vi "Mining and Dumping_r3.vi"() -> ()   [LabVIEW 2015]
uses:
  <vilib>/myRIO/Instrument Drivers/Onboard IO/PWM/typedefs/PWM Reference.ctl
  <vilib>/myRIO/Common/Instrument Driver Framework/Utilities/typedefs/myRIO Generic Hardware Reference.ctl
  <vilib>/myRIO/Common/Instrument Driver Framework/Utilities/typedefs/Hardware Version Enum.ctl
  <vilib>/myRIO/Common/Instrument Driver Framework/Utilities/typedefs/myRIO v1.0 Reference.ctl
  <vilib>/myRIO/Common/Instrument Driver Framework/Utilities/typedefs/Generic FPGA Reference.ctl
  <vilib>/myRIO/Common/Instrument Driver Framework/myRIO v1.0/PWM/typedefs/PWM Channels Enum.ctl
  <vilib>/myRIO/Instrument Drivers/Onboard IO/PWM/typedefs/PWM Configuration.ctl
  <vilib>/userdefined/High Color/nirio_resource_hc.ctl
  <vilib>/myRIO/Instrument Drivers/Onboard IO/AI/typedefs/AI Reference.ctl
  <vilib>/myRIO/Common/Instrument Driver Framework/myRIO v1.0/AI/typedefs/AI Channels List.ctl
  <vilib>/myRIO/Common/Instrument Driver Framework/myRIO v1.0/AI/typedefs/AI Channels Enum.ctl
  <vilib>/myRIO/Common/Instrument Driver Framework/Utilities/typedefs/Analog Scaling Constants List.ctl
  <vilib>/myRIO/Common/Instrument Driver Framework/Utilities/typedefs/Analog Scaling Constants.ctl
  <vilib>/myRIO/Common/Instrument Driver Framework/Utilities/vis/Is FPGA Ref Available.vi
  <vilib>/myRIO/Common/Instrument Driver Framework/myRIO v1.0/AI/vis/myRIO v1.1 Open AI.vi
  <vilib>/myRIO/Instrument Drivers/Onboard IO/AI/vis/Read.vi
  <vilib>/myRIO/Common/Instrument Driver Framework/myRIO v1.0/PWM/vis/myRIO v1.1 Open PWM.vi
  <vilib>/myRIO/Instrument Drivers/Onboard IO/PWM/vis/Set Duty Cycle and Frequency.vi
  <vilib>/myRIO/Common/Instrument Driver Framework/Utilities/vis/Validate Channels.vi
  <vilib>/myRIO/Common/Instrument Driver Framework/myRIO v1.0/AI/vis/myRIO v1.0 Reserve AI.vi
  <vilib>/myRIO/Common/Instrument Driver Framework/myRIO v1.0/PWM/vis/myRIO v1.0 Reserve PWM.vi
  <vilib>/myRIO/Common/Instrument Driver Framework/myRIO v1.0/AI/vis/myRIO v1.0 Build MUX Configuration AI.vi
  <vilib>/myRIO/Common/Instrument Driver Framework/myRIO v1.0/Resource Manager/vis/myRIO v1.0 Reserve Channel List.vi
  <vilib>/myRIO/Common/Instrument Driver Framework/myRIO v1.0/PWM/vis/myRIO v1.0 Build MUX Configuration PWM.vi
  <vilib>/myRIO/Common/Instrument Driver Framework/myRIO v1.0/Resource Manager/vis/myRIO v1.0 Reserve Channel.vi
  <vilib>/myRIO/Common/Instrument Driver Framework/myRIO v1.0/Resource Manager/vis/myRIO v1.0 Unreserve Channel.vi
  <vilib>/myRIO/Common/Instrument Driver Framework/myRIO v1.0/Resource Manager/vis/myRIO v1.0 Create Configuration List.vi
  <vilib>/myRIO/Common/Instrument Driver Framework/myRIO v1.0/Resource Manager/vis/myRIO v1.0 Build Mutex Name.vi
  <vilib>/Utility/VariantDataType/GetNumericInfo.vi
  <vilib>/Utility/error.llb/Error Cluster From Error Code.vi
  <vilib>/myRIO/Common/Instrument Driver Framework/myRIO v1.0/myRIO v1.1 Open.vi
  <vilib>/myRIO/Common/Instrument Driver Framework/Utilities/vis/IO Manager.vi
  <vilib>/myRIO/Common/Instrument Driver Framework/Utilities/vis/Configuration Manager.vi
  <vilib>/myRIO/Common/Instrument Driver Framework/myRIO v1.0/Resource Manager/vis/myRIO v1.0 Configure IO.vi
  <vilib>/myRIO/Common/Instrument Driver Framework/myRIO v1.0/myRIO v1.0 Close.vi
  <vilib>/myRIO/Common/Instrument Driver Framework/myRIO v1.0/PWM/vis/myRIO v1.0 Write PWM.vi
  <vilib>/myRIO/Common/Instrument Driver Framework/myRIO v1.0/AI/vis/myRIO v1.0 Get Scaling Constants AI.vi
  <vilib>/myRIO/Common/Instrument Driver Framework/myRIO v1.0/AI/vis/myRIO v1.0 Read AI.vi
  <vilib>/myRIO/Express VI/Onboard IO/PWM/PWM Express VI.xnode
  <vilib>/myRIO/Instrument Drivers/Onboard IO/PWM/vis/myRIO PWM Open.xnode
  <vilib>/myRIO/Express VI/Onboard IO/AI/AI Express VI.xnode
  <vilib>/myRIO/Instrument Drivers/Onboard IO/AI/vis/myRIO AI Open.xnode
  <vilib>/myRIO/Instrument Drivers/Onboard IO/PWM/PWM.lvlib
  <vilib>/myRIO/Instrument Drivers/Onboard IO/AI/AI.lvlib
panel:
  in  "Mine or Dump":i16
  out "Stop":bool
  out "Elapsed Time (s)":dbl
  out "Elapsed Time (s) 2":dbl caption="Elapsed Time (s)"
  out "Stop Dumping":bool
  out "Servo Positioin 2":dbl
  out "Servo Position 1":dbl
  out "Servo Stop":i64
  out "Stop Mining":bool
  out "DRUM IS FULL":bool
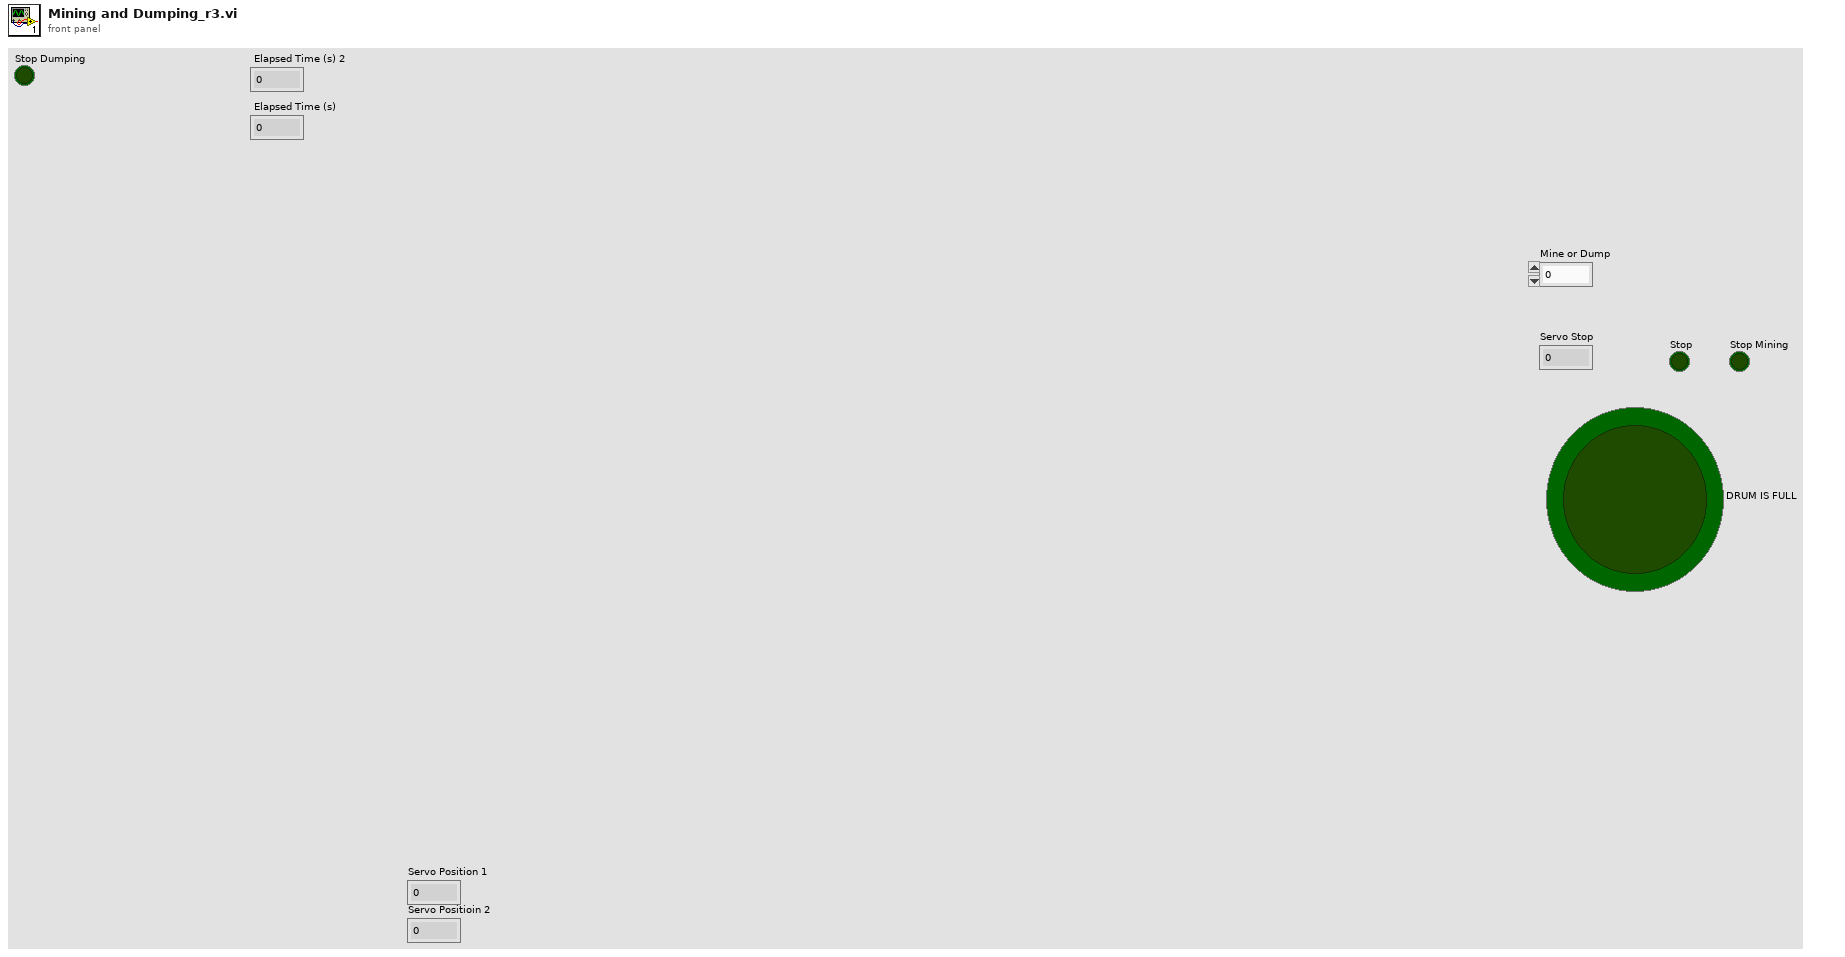
[diagram p1: front panel]
types:
  T1 = typedef "PWM.lvlib/PWM Reference.ctl" = cluster{"myRIO Reference":T2, "PWM Channels Enum":T6, "PWM Configuration":T7}
  T2 = typedef "myRIO Generic Hardware Reference.ctl" = cluster{"myRIO Model":T3, "myRIO Hardware Reference":T4}
  T3 = typedef "Hardware Version Enum.ctl" = enum16{"Unknown", "myRIO-1900", "myRIO-1950", "roboRIO"}
  T4 = typedef "myRIO v1.0 Reference.ctl" = cluster{"Generic FPGA Reference":T5, "Allow multiple opens":bool}
  T5 = typedef "Generic FPGA Reference.ctl" = refnum<k20>
  T6 = typedef "PWM Channels Enum.ctl" = enum16{"Not Connected", "C/PWM0", "C/PWM1", "A/PWM0", "A/PWM1", "A/PWM2", "B/PWM0", "B/PWM1", "B/PWM2", "PWM/PWM0", "PWM/PWM1", "PWM/PWM2", "PWM/PWM3", "PWM/PWM4", "PWM/PWM5", "PWM/PWM6", "PWM/PWM7", "PWM/PWM8", "PWM/PWM9"}
  T7 = typedef "PWM.lvlib/PWM Configuration.ctl" = cluster{"Frequency":dbl, "Duty Cycle":dbl}
  T8 = typedef "nirio_resource_hc.ctl" = tag
  T9 = typedef "AI.lvlib/AI Reference.ctl" = cluster{"myRIO Reference":T2, "AI Channels List":T10, "AI Scaling Constants List":T12}
  T10 = typedef "AI Channels List.ctl" = T11[]
  T11 = typedef "AI Channels Enum.ctl" = enum16{"Not Connected", "AudioIn/Left", "AudioIn/Right", "C/AI0", "C/AI1", "A/AI0", "A/AI1", "A/AI2", "A/AI3", "B/AI0", "B/AI1", "B/AI2", "B/AI3", "AI/AI0", "AI/AI1", "AI/AI2", "AI/AI3"}
  T12 = typedef "Analog Scaling Constants List.ctl" = T13[]
  T13 = typedef "Analog Scaling Constants.ctl" = cluster{"LSB Weight (Volts)":dbl, "Offset (Volts)":dbl, "Signed?":bool}
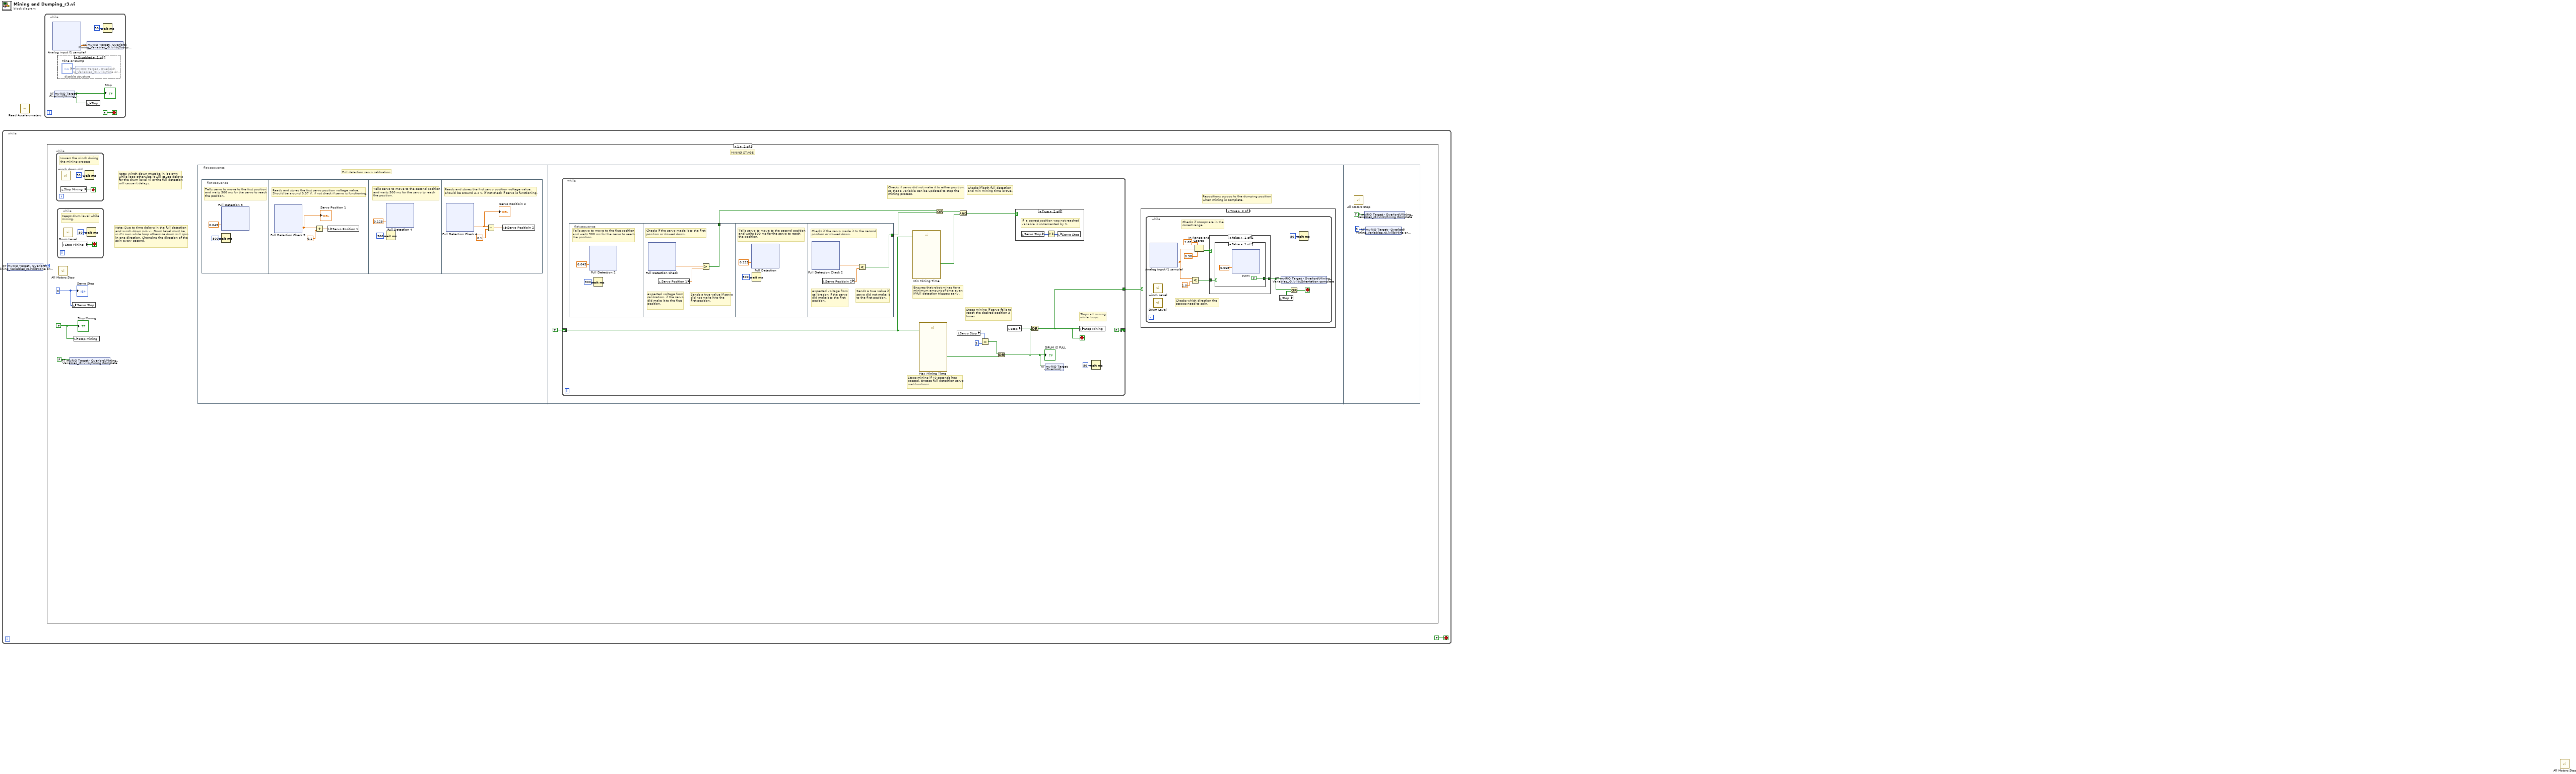
[diagram p0: block diagram]
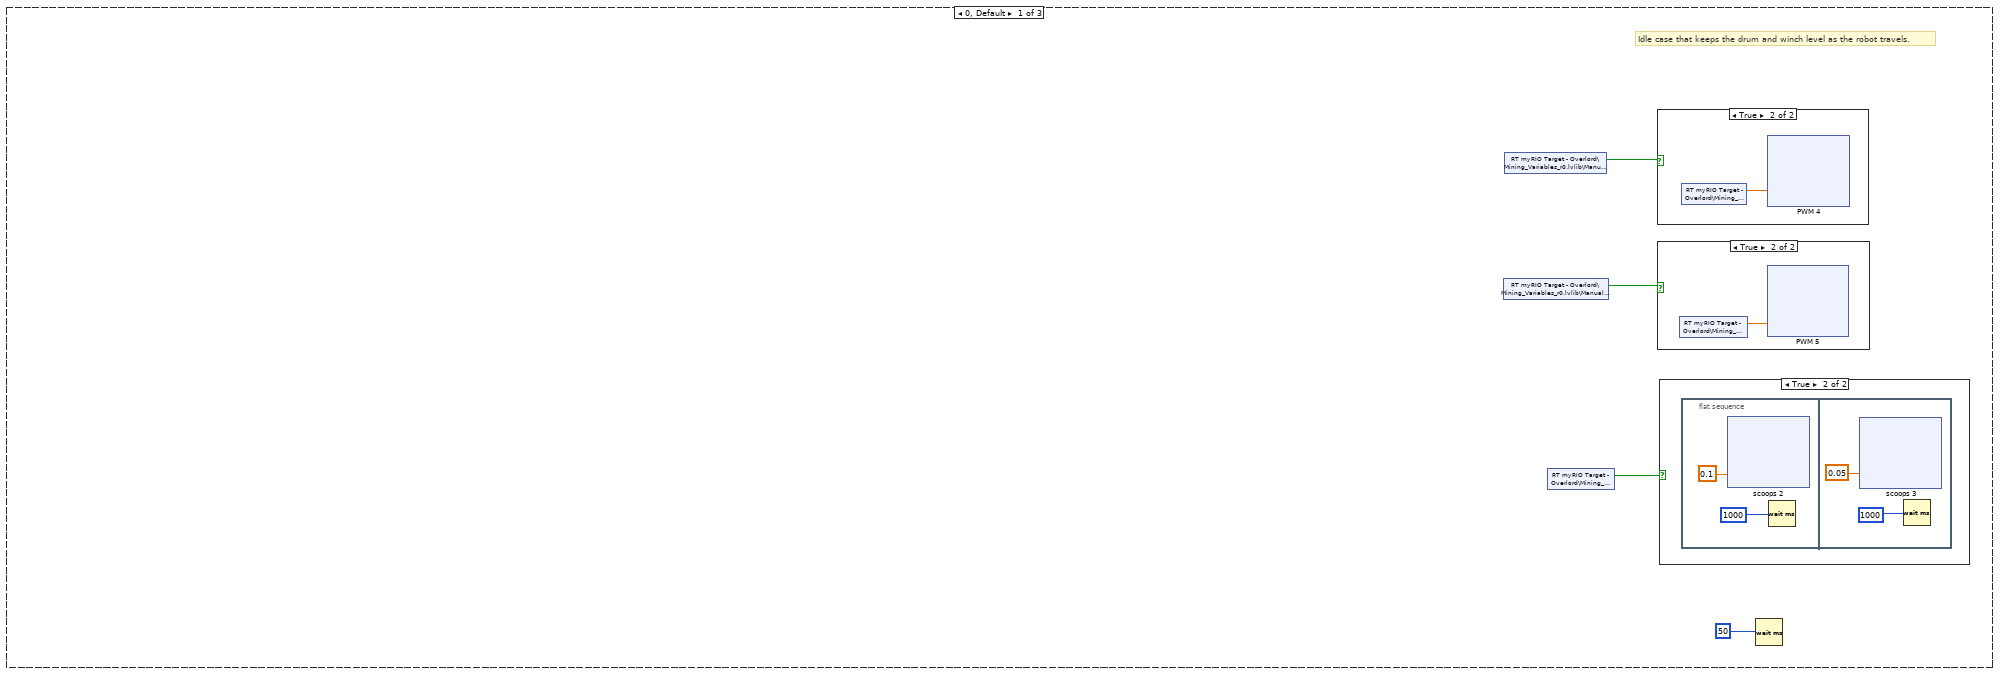
[diagram p3: hidden frame]
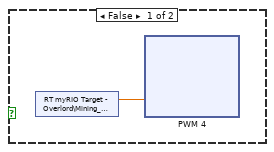
[diagram p4: hidden frame]
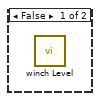
[diagram p5: hidden frame]
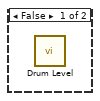
[diagram p6: hidden frame]
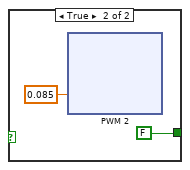
[diagram p8: hidden frame]
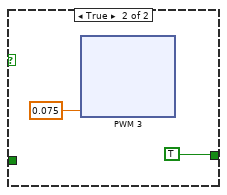
[diagram p9: hidden frame]
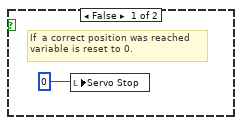
[diagram p10: hidden frame]
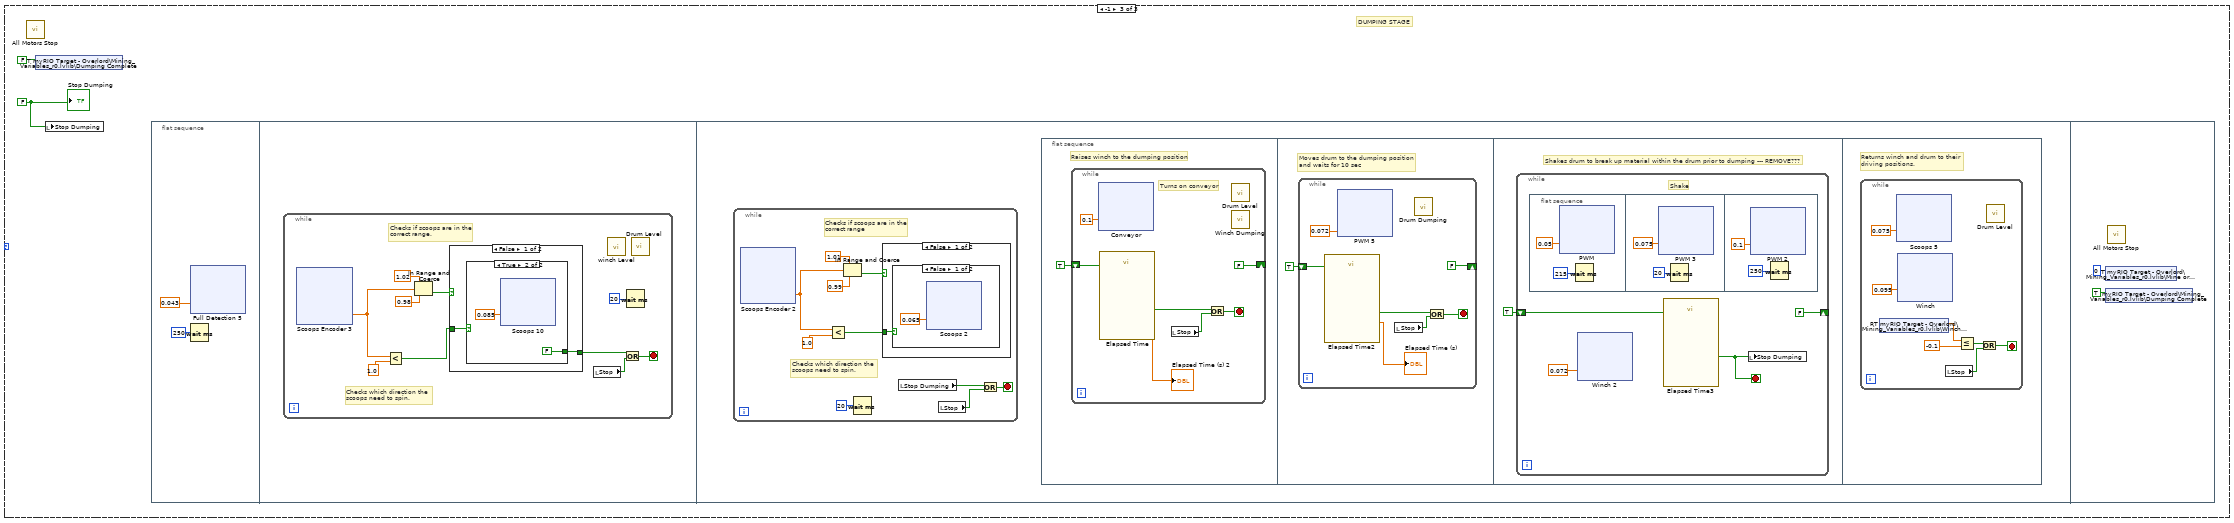
[diagram p11: hidden frame]
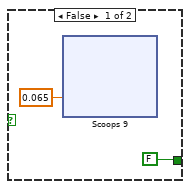
[diagram p12: hidden frame]
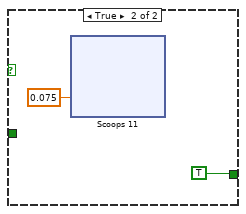
[diagram p13: hidden frame]
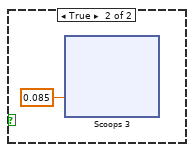
[diagram p14: hidden frame]
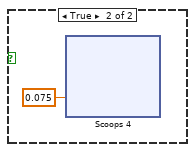
[diagram p15: hidden frame]
diagram:
  n1 = while {
    stop <- FALSE stop-if-true
    n2 = shared-variable "RT myRIO Target - Overlord\\Mining_Variables_r0.lvlib\\Mine or Dump"() -> (w1:i16)  [unwired: 1 in, 1 out]
    n3 = case shown="1" w1 {
      frame 0, Default {
        # "Idle case that keeps the drum and winch level as the robot travels."
        n4 = shared-variable "RT myRIO Target - Overlord\\Mining_Variables_r0.lvlib\\Manual Winch"() -> (w6:bool)  [unwired: 1 in, 1 out]
        n5 = shared-variable "RT myRIO Target - Overlord\\Mining_Variables_r0.lvlib\\Manual Drum"() -> (w5:bool)  [unwired: 1 in, 1 out]
        n6 = shared-variable "RT myRIO Target - Overlord\\Mining_Variables_r0.lvlib\\unjam"() -> (w3:bool)  [unwired: 1 in, 1 out]
        n7 = case shown="True" w5 {
          frame False {
            n8 = call "Drum Level.vi"() -> ()  [unwired: 12 in]
          }
          frame True {
            n9 = shared-variable "RT myRIO Target - Overlord\\Mining_Variables_r0.lvlib\\Drum"() -> (w153:dbl)  [unwired: 1 in, 1 out]
            n10 = xnode "PWM 4"("Duty Cycle"=w153) -> ()  [unwired: 1 in, 1 out]
          }
        }
        n11 = case shown="True" w6 {
          frame False {
            n12 = call "winch Level.vi"() -> ()  [unwired: 12 in]
          }
          frame True {
            n13 = shared-variable "RT myRIO Target - Overlord\\Mining_Variables_r0.lvlib\\Winch"() -> (w117:dbl)  [unwired: 1 in, 1 out]
            n14 = xnode "PWM 5"("Duty Cycle"=w117) -> ()  [unwired: 1 in, 1 out]
          }
        }
        n15 = case shown="True" w3 {
          frame False {
            n16 = shared-variable "RT myRIO Target - Overlord\\Mining_Variables_r0.lvlib\\Scoops"() -> (w7:dbl)  [unwired: 1 in, 1 out]
            n17 = xnode "PWM 4"("Duty Cycle"=w7) -> ()  [unwired: 1 in, 1 out]
          }
          frame True {
            n18 = flat-sequence {
              frame #0 {
                n19 = xnode "scoops 2"("Duty Cycle"=0.1) -> ()  [unwired: 1 in, 1 out]
                n20 = Wait (ms)(milliseconds to wait=u32 1000) -> ()  [unwired: 1 out]
              }
              frame #1 {
                n21 = xnode "scoops 3"("Duty Cycle"=0.05) -> ()  [unwired: 1 in, 1 out]
                n22 = Wait (ms)(milliseconds to wait=u32 1000) -> ()  [unwired: 1 out]
              }
            }
          }
        }
        n23 = Wait (ms)(milliseconds to wait=u32 50) -> ()  [unwired: 1 out]
      }
      frame 1 {
        w191 = FALSE ("Stop")
        w190 = i64 0 ("Servo Stop")
        # "MINING STAGE"
        # "Note: Winch down must be in it's own\nwhile loop otherwise it will cause delays\nfor the drum level vi or the full detection\nwill cause it delays."
        # "Note: Due to time delays in the full detection\nand winch down sub vi. Drum level must be\nin it's own while loop otherwise drum will spin\nin one direction. Changing the direction of the\nspin every second."
        n24 = while {
          stop <- w193 stop-if-true
          # "Lowers the winch during\nthe mining process"
          n25 = local read "Stop Mining"() -> (w193:bool)
          n26 = call "winch down old.vi"() -> ()  [unwired: 12 in]
          n27 = Wait (ms)(milliseconds to wait=u32 50) -> ()  [unwired: 1 out]
        }
        n28 = while {
          stop <- w685 stop-if-true
          # "Keeps drum level while \nmining."
          n29 = local read "Stop Mining"() -> (w685:bool)
          n30 = call "Drum Level.vi"() -> ()  [unwired: 12 in]
          n31 = Wait (ms)(milliseconds to wait=u32 50) -> ()  [unwired: 1 out]
        }
        n32 = call "All Motors Stop.vi"() -> ()  [unwired: 12 in]
        n33 = shared-variable "RT myRIO Target - Overlord\\Mining_Variables_r0.lvlib\\Mining Complete"(FALSE ("Mining Complete")) -> ()  [unwired: 1 in, 1 out]
        n34 = local write "Servo Stop"(w190) -> ()
        n35 = local write "Stop Mining"(w191) -> ()
        n36 = flat-sequence {
          frame #0 {
            # "Full detection servo calibration."
            n37 = flat-sequence {
              frame #0 {
                # "Tells servo to move to the first position\nand waits 500 ms for the servo to reach \nthe position."
                n38 = xnode "Full Detection 3"("Duty Cycle"=0.043) -> ()  [unwired: 1 in, 1 out]
                n39 = Wait (ms)(milliseconds to wait=u32 500) -> ()  [unwired: 1 out]
              }
              frame #1 {
                # "Reads and stores the first servo position voltage value. \nShould be around 0.97 V. if not check if servo is functioning."
                n40 = xnode "Full Detection Check 3"() -> ("A/AI0 (Pin 3)"=w232:dbl)  [unwired: 1 in, 1 out]
                "Servo Position 1" <- w232
                n41 = Add(x=w232, y=0.1) -> (x+y=w233:dbl)
                n42 = local write "Servo Position 1"(w233) -> ()
              }
              frame #2 {
                # "Tells servo to move to the second position\nand waits 500 ms for the servo to reach \nthe position."
                n43 = xnode "Full Detection 4"("Duty Cycle"=0.125) -> ()  [unwired: 1 in, 1 out]
                n44 = Wait (ms)(milliseconds to wait=u32 500) -> ()  [unwired: 1 out]
              }
              frame #3 {
                # "Reads and stores the first servo position voltage value. \nShould be around 2.4 V. if not check if servo is functioning."
                n45 = xnode "Full Detection Check 4"() -> ("A/AI0 (Pin 3)"=w309:dbl)  [unwired: 1 in, 1 out]
                "Servo Positioin 2" <- w309
                n46 = Subtract(x=w309, y=0.1) -> (x-y=w310:dbl)
                n47 = local write "Servo Positioin 2"(w310) -> ()
              }
            }
          }
          frame #1 {
            # "Repositions scoops to the dumping position\nwhen mining is complete."
            n48 = while {
              tunnel: [w515] -> w348
              shift-right: [FALSE] -> _
              shift-left: TRUE -> [w518]
              stop <- w515 stop-if-true
              # "Checks if servo did not make it to either position,\nso that a variable can be updated to stop the \nmining process."
              # "Stops all mining \nwhile loops."
              # "Stops mining if 40 seconds has \npassed. Encase full detedtion servo \nmalifunctions."
              # "Stops mining if servo fails to \nreach the desired position 3\ntimes."
              # "Checks if both full detection \nand min mining time is true."
              # "Ensures that robot mines for a \nminimum amount of time even\nif full detection triggers early."
              n49 = flat-sequence {
                tunnel: [w567] -> w513
                tunnel: [w643] -> w512
                frame #0 {
                  # "Tells servo to move to the first position\nand waits 500 ms for the servo to reach \nthe position."
                  n50 = xnode "Full Detection 2"("Duty Cycle"=0.043) -> ()  [unwired: 1 in, 1 out]
                  n51 = Wait (ms)(milliseconds to wait=u32 500) -> ()  [unwired: 1 out]
                }
                frame #1 {
                  # "Sends a true value if servo\ndid not make it to the\nfirst position."
                  # "expected voltage from \ncalibration. if the servo\ndid make it to the first \nposition."
                  # "Checks if the servo made it to the first \nposition or slowed down."
                  n52 = xnode "Full Detection Check"() -> ("A/AI0 (Pin 3)"=w566:dbl)  [unwired: 1 in, 1 out]
                  n53 = local read "Servo Position 1"() -> (w565:dbl)
                  n54 = Greater?(x=w566, y=w565) -> (0:w567:bool)
                }
                frame #2 {
                  # "Tells servo to move to the second position\nand waits 500 ms for the servo to reach \nthe position."
                  n55 = xnode "Full Detection"("Duty Cycle"=0.125) -> ()  [unwired: 1 in, 1 out]
                  n56 = Wait (ms)(milliseconds to wait=u32 500) -> ()  [unwired: 1 out]
                }
                frame #3 {
                  # "Sends a true value if\nservo did not make it\nto the first position."
                  # "expected voltage from \ncalibration if the servo\ndid makeit to the first \nposition."
                  # "Checks if the servo made it to the second \nposition or slowed down."
                  n57 = xnode "Full Detection Check 2"() -> ("A/AI0 (Pin 3)"=w644:dbl)  [unwired: 1 in, 1 out]
                  n58 = local read "Servo Positioin 2"() -> (w642:dbl)
                  n59 = Less?(x=w644, y=w642) -> (x < y?=w643:bool)
                }
              }
              n60 = call "Min Mining Time"("Reset"=w518) -> ("Time has Elapsed"=w520:bool)  [unwired: 11 in, 7 out]
              n61 = call "Max Mining Time"("Reset"=w518) -> ("Time has Elapsed"=w523:bool)  [unwired: 11 in, 7 out]
              n62 = Or(x=w513, y=w512) -> (x .or. y?=w517:bool)
              n63 = local read "Servo Stop"() -> (w524:i64)
              n64 = And(x=w517, y=w520) -> (x .and. y?=w521:bool)
              n65 = Equal?(x=w524, y=i64 3) -> (x = y?=w522:bool)
              n66 = Or(x=w522, y=w523) -> (x .or. y?=w510:bool)
              "DRUM IS FULL" <- w510
              n67 = local read "Stop"() -> (w511:bool)
              n68 = case shown="True" w521 {
                frame False {
                  # "If  a correct position was reached \nvariable is reset to 0."
                  n69 = local write "Servo Stop"(i64 0 ("Servo Stop")) -> ()
                }
                frame True {
                  # "If  a correct position was not reached \nvariable is incremented by 1."
                  n70 = local read "Servo Stop"() -> (w527:i64)
                  n71 = Increment(x=w527) -> (x+1=w526:i64)
                  n72 = local write "Servo Stop"(w526) -> ()
                }
              }
              n73 = Or(x=w511, y=w510) -> (x .or. y?=w515:bool)
              n74 = shared-variable "RT myRIO Target - Overlord\\Mining_Variables_r0.lvlib\\Full"(w510) -> ()  [unwired: 1 in, 1 out]
              n75 = local write "Stop Mining"(w515) -> ()
              n76 = Wait (ms)(milliseconds to wait=u32 50) -> ()  [unwired: 1 out]
            }
            n77 = case shown="True" w348 {
              frame False {
              }
              frame True {
                n78 = while {
                  stop <- w353 stop-if-true
                  # "Checks which direction the \nscoops need to spin."
                  # "Checks if scoops are in the\ncorrect range"
                  n79 = xnode "Analog input (1 sample)"() -> ("A/AI1 (Pin 5)"=w356:dbl)  [unwired: 1 in, 1 out]
                  n80 = call "winch Level.vi"() -> ()  [unwired: 12 in]
                  n81 = call "Drum Level.vi"() -> ()  [unwired: 12 in]
                  n82 = Less?(x=w356, y=1.0) -> (x < y?=w358:bool)
                  n83 = In Range and Coerce(upper limit=1.02, x=w356, lower limit=0.98) -> (In Range?=w357:bool)  [unwired: 1 out]
                  n84 = case shown="False" w357 {
                    tunnel: w358 -> [w361 _]
                    tunnel: [w360 TRUE] -> w350
                    frame False {
                      n85 = case shown="False" w361 {
                        tunnel: [FALSE FALSE] -> w360
                        frame False {
                          n86 = xnode "PWM"("Duty Cycle"=0.065) -> ()  [unwired: 1 in, 1 out]
                        }
                        frame True {
                          n87 = xnode "PWM 2"("Duty Cycle"=0.085) -> ()  [unwired: 1 in, 1 out]
                        }
                      }
                    }
                    frame True {
                      n88 = xnode "PWM 3"("Duty Cycle"=0.075) -> ()  [unwired: 1 in, 1 out]
                    }
                  }
                  n89 = local read "Stop"() -> (w352:bool)
                  n90 = shared-variable "RT myRIO Target - Overlord\\Mining_Variables_r0.lvlib\\Orientation complete"(w350) -> ()  [unwired: 1 in, 1 out]
                  n91 = Or(x=w350, y=w352) -> (x .or. y?=w353:bool)
                  n92 = Wait (ms)(milliseconds to wait=u32 50) -> ()  [unwired: 1 out]
                }
              }
            }
          }
          frame #2 {
            n93 = call "All Motors Stop.vi"() -> ()  [unwired: 12 in]
            n94 = shared-variable "RT myRIO Target - Overlord\\Mining_Variables_r0.lvlib\\Mining Complete"(TRUE ("Mining Complete")) -> ()  [unwired: 1 in, 1 out]
            n95 = shared-variable "RT myRIO Target - Overlord\\Mining_Variables_r0.lvlib\\Mine or Dump"(i16 0 ("Mine or Dump")) -> ()  [unwired: 1 in, 1 out]
          }
        }
        "Stop Mining" <- w191
        "Servo Stop" <- w190
      }
      frame -1 {
        w687 = FALSE
        # "DUMPING STAGE"
        n96 = call "All Motors Stop.vi"() -> ()  [unwired: 12 in]
        n97 = shared-variable "RT myRIO Target - Overlord\\Mining_Variables_r0.lvlib\\Dumping Complete"(FALSE ("Dumping Complete")) -> ()  [unwired: 1 in, 1 out]
        n98 = local write "Stop Dumping"(w687) -> ()
        n99 = flat-sequence {
          frame #0 {
            n100 = xnode "Full Detection 5"("Duty Cycle"=0.043) -> ()  [unwired: 1 in, 1 out]
            n101 = Wait (ms)(milliseconds to wait=u32 250) -> ()  [unwired: 1 out]
          }
          frame #1 {
            n102 = while {
              stop <- w728 stop-if-true
              # "Checks which direction the \nscoops need to spin."
              # "Checks if scoops are in the\ncorrect range."
              n103 = xnode "Scoops Encoder 3"() -> ("A/AI1 (Pin 5)"=w731:dbl)  [unwired: 1 in, 1 out]
              n104 = Less?(x=w731, y=1.0) -> (x < y?=w729:bool)
              n105 = In Range and Coerce(upper limit=1.02, x=w731, lower limit=0.98) -> (In Range?=w730:bool)  [unwired: 1 out]
              n106 = case shown="False" w730 {
                tunnel: w729 -> [w736 _]
                tunnel: [w735 TRUE] -> w727
                frame False {
                  n107 = case shown="True" w736 {
                    tunnel: [FALSE FALSE] -> w735
                    frame False {
                      n108 = xnode "Scoops 9"("Duty Cycle"=0.065) -> ()  [unwired: 1 in, 1 out]
                    }
                    frame True {
                      n109 = xnode "Scoops 10"("Duty Cycle"=0.085) -> ()  [unwired: 1 in, 1 out]
                    }
                  }
                }
                frame True {
                  n110 = xnode "Scoops 11"("Duty Cycle"=0.075) -> ()  [unwired: 1 in, 1 out]
                }
              }
              n111 = local read "Stop"() -> (w726:bool)
              n112 = call "winch Level.vi"() -> ()  [unwired: 12 in]
              n113 = Or(x=w727, y=w726) -> (x .or. y?=w728:bool)
              n114 = Wait (ms)(milliseconds to wait=u32 20) -> ()  [unwired: 1 out]
              n115 = call "Drum Level.vi"() -> ()  [unwired: 12 in]
            }
          }
          frame #2 {
            n116 = while {
              stop <- w888 stop-if-true
              # "Checks which direction the \nscoops need to spin."
              # "Checks if scoops are in the\ncorrect range"
              n117 = xnode "Scoops Encoder 2"() -> ("A/AI1 (Pin 5)"=w891:dbl)  [unwired: 1 in, 1 out]
              n118 = Less?(x=w891, y=1.0) -> (x < y?=w893:bool)
              n119 = In Range and Coerce(upper limit=1.01, x=w891, lower limit=0.99) -> (In Range?=w892:bool)  [unwired: 1 out]
              n120 = Wait (ms)(milliseconds to wait=u32 20) -> ()  [unwired: 1 out]
              n121 = case shown="False" w892 {
                tunnel: w893 -> [w895 _]
                frame False {
                  n122 = case shown="False" w895 {
                    frame False {
                      n123 = xnode "Scoops 2"("Duty Cycle"=0.065) -> ()  [unwired: 1 in, 1 out]
                    }
                    frame True {
                      n124 = xnode "Scoops 3"("Duty Cycle"=0.085) -> ()  [unwired: 1 in, 1 out]
                    }
                  }
                }
                frame True {
                  n125 = xnode "Scoops 4"("Duty Cycle"=0.075) -> ()  [unwired: 1 in, 1 out]
                }
              }
              n126 = local read "Stop Dumping"() -> (w886:bool)
              n127 = local read "Stop"() -> (w887:bool)
              n128 = Or(x=w886, y=w887) -> (x .or. y?=w888:bool)
            }
            n129 = flat-sequence {
              frame #0 {
                # "Raises winch to the dumping position"
                n130 = while {
                  shift-right: [FALSE ("Reset")] -> _
                  shift-left: TRUE ("Reset") -> [w1044]
                  stop <- w1047 stop-if-true
                  # "Turns on conveyor"
                  n131 = xnode "Conveyor"("Duty Cycle"=0.1) -> ()  [unwired: 1 in, 1 out]
                  n132 = call "Elapsed Time"("Reset"=w1044) -> ("Elapsed Time (s)"=→"Elapsed Time (s) 2":dbl, "Time has Elapsed"=w1042:bool)  [unwired: 11 in, 6 out]
                  n133 = local read "Stop"() -> (w1046:bool)
                  n134 = Or(x=w1042, y=w1046) -> (x .or. y?=w1047:bool)
                  n135 = call "Drum Level.vi"() -> ()  [unwired: 12 in]
                  n136 = call "Winch Dumping.vi"() -> ()  [unwired: 12 in]
                }
              }
              frame #1 {
                # "Moves drum to the dumping position\nand waits for 10 sec"
                n137 = while {
                  shift-right: [FALSE ("Reset")] -> _
                  shift-left: TRUE ("Reset") -> [w1086]
                  stop <- w1091 stop-if-true
                  n138 = call "Elapsed Time2"("Reset"=w1086) -> ("Elapsed Time (s)"=→"Elapsed Time (s)":dbl, "Time has Elapsed"=w1090:bool)  [unwired: 11 in, 6 out]
                  n139 = xnode "PWM 5"("Duty Cycle"=0.072) -> ()  [unwired: 1 in, 1 out]
                  n140 = local read "Stop"() -> (w1089:bool)
                  n141 = call "Drum Dumping.vi"() -> ()  [unwired: 12 in]
                  n142 = Or(x=w1090, y=w1089) -> (x .or. y?=w1091:bool)
                }
              }
              frame #2 {
                # "Shakes drum to break up material within the drum prior to dumping --- REMOVE???"
                n143 = while {
                  shift-right: [FALSE] -> _
                  shift-left: TRUE -> [w1130]
                  stop <- w1128 stop-if-true
                  # "Shake"
                  n144 = flat-sequence {
                    frame #0 {
                      n145 = xnode "PWM"("Duty Cycle"=0.05) -> ()  [unwired: 1 in, 1 out]
                      n146 = Wait (ms)(milliseconds to wait=u32 215) -> ()  [unwired: 1 out]
                    }
                    frame #1 {
                      n147 = xnode "PWM 3"("Duty Cycle"=0.075) -> ()  [unwired: 1 in, 1 out]
                      n148 = Wait (ms)(milliseconds to wait=u32 20) -> ()  [unwired: 1 out]
                    }
                    frame #2 {
                      n149 = xnode "PWM 2"("Duty Cycle"=0.1) -> ()  [unwired: 1 in, 1 out]
                      n150 = Wait (ms)(milliseconds to wait=u32 250) -> ()  [unwired: 1 out]
                    }
                  }
                  n151 = xnode "Winch 2"("Duty Cycle"=0.072) -> ()  [unwired: 1 in, 1 out]
                  n152 = call "Elapsed Time3"("Reset"=w1130) -> ("Time has Elapsed"=w1128:bool)  [unwired: 11 in, 7 out]
                  n153 = local write "Stop Dumping"(w1128) -> ()
                }
              }
              frame #3 {
                # "Returns winch and drum to their \ndriving positions."
                n154 = while {
                  stop <- w1280 stop-if-true
                  n155 = shared-variable "RT myRIO Target - Overlord\\Mining_Variables_r0.lvlib\\Winch Accel x"() -> (w1279:dbl)  [unwired: 1 in, 1 out]
                  n156 = xnode "Scoops 5"("Duty Cycle"=0.075) -> ()  [unwired: 1 in, 1 out]
                  n157 = xnode "Winch"("Duty Cycle"=0.095) -> ()  [unwired: 1 in, 1 out]
                  n158 = local read "Stop"() -> (w1281:bool)
                  n159 = Less Or Equal?(x=w1279, y=-0.1) -> (x <= y?=w1282:bool)
                  n160 = Or(x=w1282, y=w1281) -> (x .or. y?=w1280:bool)
                  n161 = call "Drum Level.vi"() -> ()  [unwired: 12 in]
                }
              }
            }
          }
          frame #3 {
            n162 = shared-variable "RT myRIO Target - Overlord\\Mining_Variables_r0.lvlib\\Dumping Complete"(TRUE ("Dumping Complete")) -> ()  [unwired: 1 in, 1 out]
            n163 = shared-variable "RT myRIO Target - Overlord\\Mining_Variables_r0.lvlib\\Mine or Dump"(i16 0 ("Mine or Dump")) -> ()  [unwired: 1 in, 1 out]
            n164 = call "All Motors Stop.vi"() -> ()  [unwired: 12 in]
          }
        }
        "Stop Dumping" <- w687
      }
    }
  }
  n165 = call "Read Accelerometers.vi"() -> ()  [unwired: 11 in, 9 out]
  n166 = while {
    stop <- FALSE stop-if-true
    n167 = xnode "Analog input (1 sample)"() -> ("A/AI1 (Pin 5)"=w1358:dbl)  [unwired: 1 in, 1 out]
    n168 = shared-variable "RT myRIO Target - Overlord\\Mining_Variables_r0.lvlib\\Stop"() -> (w1359:bool)  [unwired: 1 in, 1 out]
    "Stop" <- w1359
    n169 = disable-structure shown="Disabled" {
      frame Disabled {
        n170 = shared-variable "RT myRIO Target - Overlord\\Mining_Variables_r0.lvlib\\Mine or Dump"("Mine or Dump") -> ()  [unwired: 1 in, 1 out]
      }
      frame Enabled {
      }
    }
    n171 = local write "Stop"(w1359) -> ()
    n172 = shared-variable "RT myRIO Target - Overlord\\Mining_Variables_r0.lvlib\\Scoop Position"(w1358) -> ()  [unwired: 1 in, 1 out]
    n173 = Wait (ms)(milliseconds to wait=u32 50) -> ()  [unwired: 1 out]
  }
  n174 = call "All Motors Stop.vi"() -> ()  [unwired: 12 in]
